vi "TestRFGVComplete.vi"() -> (0 "error out":errorcluster, 2 "Pass":bool)   [LabVIEW 2015]
uses:
  TypeDef/RequestActionEnum.ctl
  LVClasses/Request/PersonnelType.ctl
  TypeDef/PersonnelAndTime.ctl
  LVClasses/Request/Request.lvclass/Request.ctl
  LVClasses/Request/Read FulfilledName.vi
  LVClasses/Request/Read FulfilledTime.vi
  LVClasses/Request/Request.lvclass
panel:
  out "TimeStamp":bool
  out "Name":bool
  out "Request":string
  out "Add Request":string
  out "Ack":string
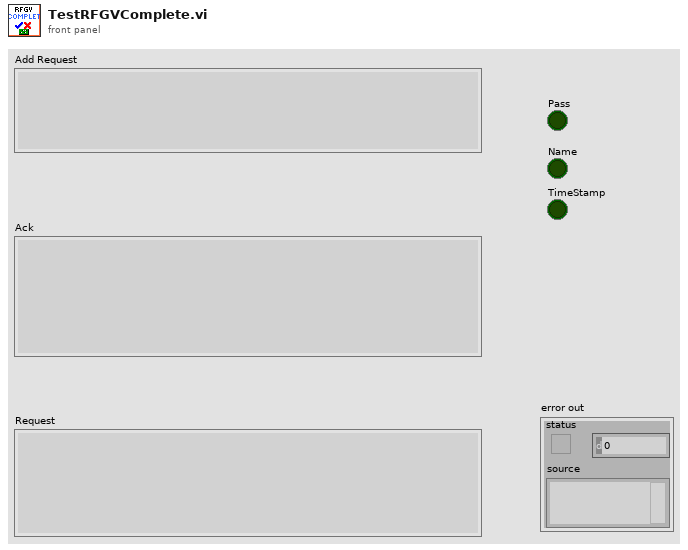
[diagram p1: front panel]
types:
  T1 = typedef "PersonnelAndTime.ctl" = cluster{"Personnel":string, "TimeStamp":string}
  T2 = typedef "RequestActionEnum.ctl" = enum16{"Init", "ReadRequests", "ReadRequest", "AddRequest", "RemoveRequest", "ToDisk", "Ack", "Complete", "Read Summary"}
  T3 = typedef "Request.lvclass/PersonnelType.ctl" = enum16{"Nurse", "Doctor", "Cleanning", "Admin"}
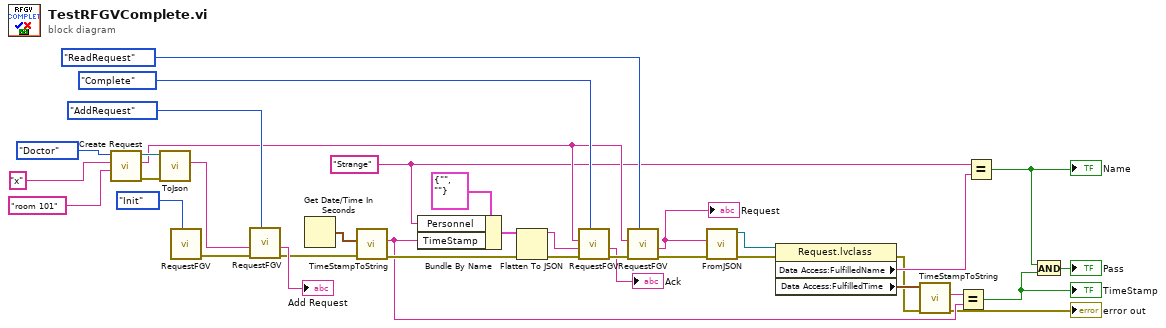
[diagram p0: block diagram]
diagram:
  w7 = "Strange" ("Personnel")
  n1 = call "Create Request.vi"(".Description"="room 101" (".Description 2"), "Name"="x" ("Name 2"), "Personnel Type"=PersonnelType."Doctor" ("Type 2")) -> ("error out"=w34:errorcluster, "RUID"=w14:string, "Request out"=w33:refnum<class "Request.lvclass">)  [unwired: 6 in]
  n2 = call "ToJson.vi"("error in (no error)"=w34, "Request"=w33) -> ("Request"=w32:string)  [unwired: 8 in, 1 out]
  n3 = call "RequestFGV.vi"("Actions"=RequestActionEnum."Init") -> ("error out"=w26:errorcluster)  [unwired: 9 in, 1 out]
  n4 = call "RequestFGV.vi"("Actions"=RequestActionEnum."AddRequest", "error in (no error)"=w26, "Data In"=w32) -> ("error out"=w16:errorcluster, "Data Out"=→"Add Request":string)  [unwired: 7 in]
  n5 = Get Date/Time In Seconds() -> (seconds since 1Jan1904=w22:timestamp)
  n6 = call "TimeStampToString.vi"("error in (no error)"=w16, "Time Stamp"=w22) -> ("error out"=w18:errorcluster, "String"=w9:string)  [unwired: 8 in]
  n7 = Bundle By Name(cluster=T1 {"Personnel"="", "TimeStamp"=""}, "Personnel"=w7, "TimeStamp"=w9) -> (w21:T1)
  n8 = Flatten To JSON(anything=w21, error in (no error)=w18) -> (JSON string=w20:string, 11:w19:errorcluster)  [unwired: 1 in]
  n9 = call "RequestFGV.vi"("Actions"=RequestActionEnum."Complete", "error in (no error)"=w19, "Data In"=w20, "RUID"=w14) -> ("error out"=w24:errorcluster, "Data Out"=→"Ack":string)  [unwired: 6 in]
  n10 = call "RequestFGV.vi"("Actions"=RequestActionEnum."ReadRequest", "error in (no error)"=w24, "RUID"=w14) -> ("error out"=w15:errorcluster, "Data Out"=w13:string)  [unwired: 7 in]
  "Request" <- w13
  n11 = call "FromJSON.vi"("error in (no error)"=w15, "Request"=w13) -> ("error out"=w3:errorcluster, "Request out"=w12:refnum<class "Request.lvclass">)  [unwired: 8 in]
  n12 = property class="Request.lvclass"(reference=w12, error in=w3) -> (error out=w2:errorcluster, "Data Access:FulfilledName"=w8:string, "Data Access:FulfilledTime"=w11:timestamp)  [unwired: 1 out]
  n13 = call "TimeStampToString.vi"("error in (no error)"=w2, "Time Stamp"=w11) -> ("error out"=→"error out":errorcluster, "String"=w10:string)  [unwired: 8 in]
  n14 = Equal?(x=w10, y=w9) -> (x = y?=w5:bool)
  "TimeStamp" <- w5
  n15 = Equal?(x=w7, y=w8) -> (x = y?=w6:bool)
  "Name" <- w6
  n16 = And(x=w6, y=w5) -> (x .and. y?=→"Pass":bool)
